vi "Calibration-Frame6.vi"() -> (1 "String":string, 2 "String 2":string, 3 "Boolean":bool, 4 "Array":string[](array[string]), 5 "Boolean 2":bool, 6 "Boolean 3":bool)   [LabVIEW 2015]
uses:
  Anemometry Sub Vis/Globals/Calib_global.vi
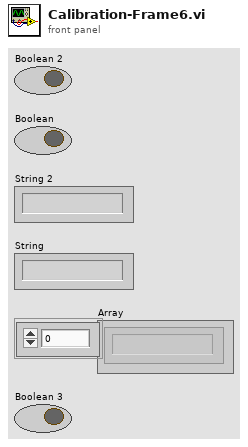
[diagram p1: front panel]
types:
  T1 = typedef "Ref_Inst_type.ctl" = enum16{"Propellor anemometer", "Pressure Transducer", "Raw voltage", "Pitot-static tube", "Preston tube", "Generic Linear", "Generic Polynomial", "Thermocouple", "LDA", "Enter Value", "ADAM Channel"}
  T2 = typedef "Cal_Inst_type.ctl" = enum16{"Propeller anemometer", "Pressure Transducer", "Hot wire", "Cross wire velocity", "Cross wire angle", "Generic Linear", "Generic Polynomial", "Generic BackPoly", "Fast FID", "Thermocouple", "Cold wire", "Pulsed Wire"}
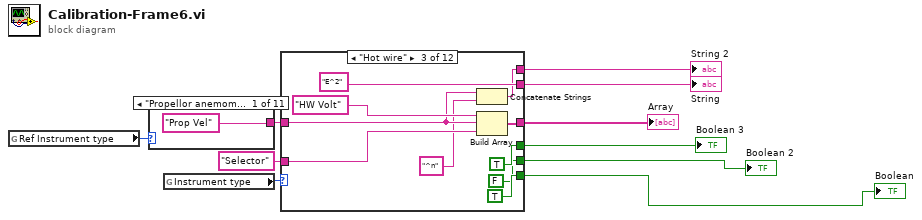
[diagram p0: block diagram]
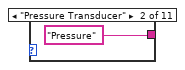
[diagram p2: hidden frame]
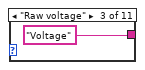
[diagram p3: hidden frame]
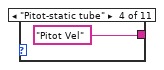
[diagram p4: hidden frame]
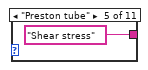
[diagram p5: hidden frame]
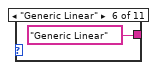
[diagram p6: hidden frame]
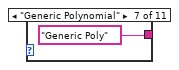
[diagram p7: hidden frame]
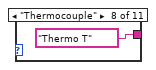
[diagram p8: hidden frame]
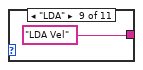
[diagram p9: hidden frame]
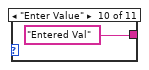
[diagram p10: hidden frame]
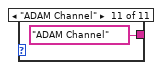
[diagram p11: hidden frame]
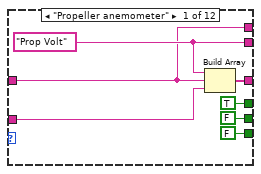
[diagram p12: hidden frame]
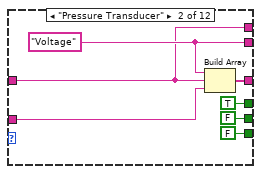
[diagram p13: hidden frame]
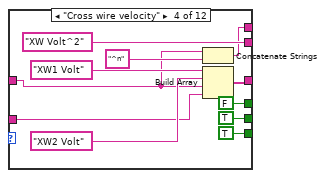
[diagram p14: hidden frame]
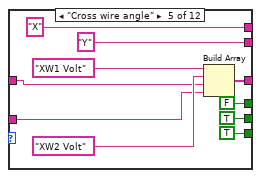
[diagram p15: hidden frame]
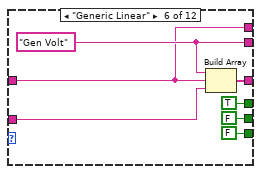
[diagram p16: hidden frame]
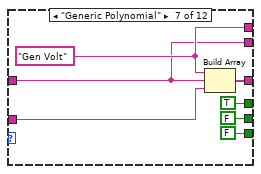
[diagram p17: hidden frame]
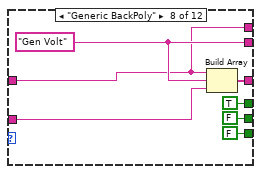
[diagram p18: hidden frame]
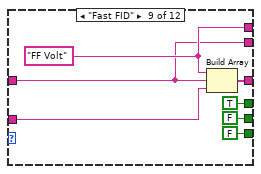
[diagram p19: hidden frame]
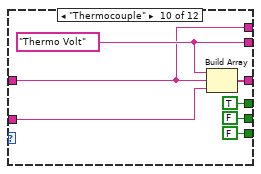
[diagram p20: hidden frame]
diagram:
  n1 = global read "Calib_global.vi" "Ref Instrument type"() -> (w7:T1)
  n2 = case shown="\"Propellor anemometer\"" w7 {
    tunnel: ["Prop Vel" "Pressure" "Voltage" "Pitot Vel" "Shear stress" "Generic Linear" "Generic Poly" "Thermo T" "LDA Vel" "Entered Val" "ADAM Channel"] -> w4
    frame "Propellor anemometer" {
    }
    frame "Pressure Transducer" {
    }
    frame "Raw voltage" {
    }
    frame "Pitot-static tube" {
    }
    frame "Preston tube" {
    }
    frame "Generic Linear" {
    }
    frame "Generic Polynomial" {
    }
    frame "Thermocouple" {
    }
    frame "LDA" {
    }
    frame "Enter Value" {
    }
    frame "ADAM Channel" {
    }
  }
  n3 = global read "Calib_global.vi" "Instrument type"() -> (w6:T2)
  n4 = case shown="\"Hot wire\"" w6 {
    tunnel: [FALSE FALSE TRUE TRUE TRUE FALSE FALSE FALSE FALSE FALSE FALSE FALSE] -> w10
    tunnel: [TRUE TRUE TRUE FALSE FALSE TRUE TRUE TRUE TRUE TRUE TRUE TRUE] -> w2
    tunnel: [FALSE FALSE FALSE TRUE TRUE FALSE FALSE FALSE FALSE FALSE FALSE FALSE] -> w3
    tunnel: w4 -> [w22 w29 w38 w48 w58 w68 w74 w81 w88 w96 w102 w109]
    tunnel: [w25 w32 w41 w51 w61 w70 w77 w84 w91 w98 w105 w112] -> w5
    tunnel: "Selector" -> [w24 w31 w40 w50 w60 w67 w76 w83 w90 w95 w104 w111]
    tunnel: [w23 w30 "E^2" "XW Volt^2" "Y" w69 w74 w82 w88 w97 w102 w109] -> w9
    tunnel: [w22 w29 w36 w46 "X" w68 w75 w81 w89 w96 w103 w110] -> w8
    frame "Propeller anemometer" {
      w23 = "Prop Volt"
      n5 = Build Array(w23, w22, w24) -> (w25:string[])
    }
    frame "Pressure Transducer" {
      w30 = "Voltage"
      n6 = Build Array(w30, w29, w31) -> (w32:string[])
    }
    frame "Hot wire" {
      n7 = Concatenate Strings(w38, "^n") -> (w36:string)
      n8 = Build Array("HW Volt", w38, w40) -> (w41:string[])
    }
    frame "Cross wire velocity" {
      n9 = Concatenate Strings(w48, "^n") -> (w46:string)
      n10 = Build Array("XW1 Volt", "XW2 Volt", w48, w50) -> (w51:string[])
    }
    frame "Cross wire angle" {
      n11 = Build Array("XW1 Volt", "XW2 Volt", w58, w60) -> (w61:string[])
    }
    frame "Generic Linear" {
      w69 = "Gen Volt"
      n12 = Build Array(w69, w68, w67) -> (w70:string[])
    }
    frame "Generic Polynomial" {
      w75 = "Gen Volt"
      n13 = Build Array(w75, w74, w76) -> (w77:string[])
    }
    frame "Generic BackPoly" {
      w82 = "Gen Volt"
      n14 = Build Array(w81, w82, w83) -> (w84:string[])
    }
    frame "Fast FID" {
      w89 = "FF Volt"
      n15 = Build Array(w89, w88, w90) -> (w91:string[])
    }
    frame "Thermocouple" {
      w97 = "Thermo Volt"
      n16 = Build Array(w97, w96, w95) -> (w98:string[])
    }
    frame "Cold wire" {
      w103 = "CW Volt"
      n17 = Build Array(w103, w102, w104) -> (w105:string[])
    }
    frame "Pulsed Wire" {
      w110 = "1/TOF"
      n18 = Build Array(w110, w109, w111) -> (w112:string[])
    }
  }
  "Boolean" <- w10
  "String" <- w9
  "String 2" <- w8
  "Array" <- w5
  "Boolean 2" <- w3
  "Boolean 3" <- w2
